vi "verify communication.vi"(8 "error in (no error)":errorcluster, 11 "Server in":refnum<class "Server.lvclass">) -> (0 "error out":errorcluster, 3 "Server out":refnum<class "Server.lvclass">)   [LabVIEW 2018, in "Server.lvclass"]
uses:
  Server.lvclass
  Server.lvclass/Server.ctl
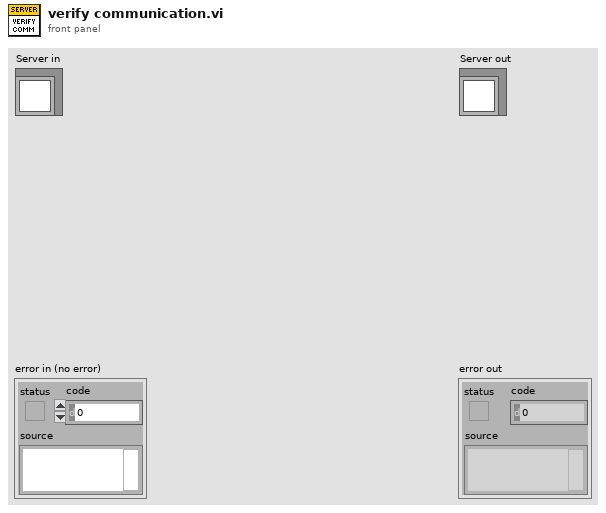
[diagram p1: front panel]
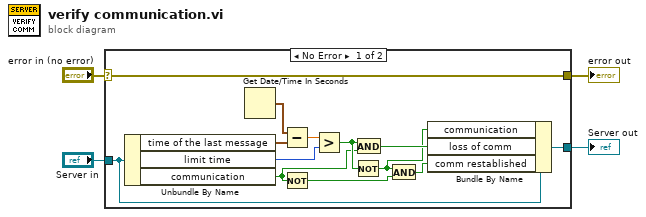
[diagram p0: block diagram]
diagram:
  n1 = case shown="No Error" "error in (no error)" {
    selector: "error in (no error)" -> [w17 w19]
    tunnel: [w17 w19] -> w3
    tunnel: [w11 w18] -> w1
    tunnel: "Server in" -> [w12 w18]
    frame No Error {
      n2 = Unbundle By Name(w12) -> ("time of the last message"=w15:timestamp, "limit time"=w13:u16, "communication"=w7:bool)
      n3 = Get Date/Time In Seconds() -> (seconds since 1Jan1904=w16:timestamp)
      n4 = Subtract(x=w16, y=w15) -> (x-y=w14:dbl)
      n5 = Not(x=w7) -> (.not. x?=w6:bool)
      n6 = Greater?(x=w14, y=w13) -> (0:w9:bool)
      n7 = Not(x=w9) -> (.not. x?=w5:bool)
      n8 = And(x=w9, y=w7) -> (x .and. y?=w10:bool)
      n9 = And(x=w5, y=w6) -> (x .and. y?=w8:bool)
      n10 = Bundle By Name(cluster=w12, "communication"=w5, "loss of comm"=w10, "comm restablished"=w8) -> (w11:refnum<class "Server.lvclass">)
    }
    frame Error {
    }
  }
  "error out" <- w3
  "Server out" <- w1
